vi "CalculateIrradiance.vi"(0 "Base Irradiance µW/cm²":dbl, 1 "Array":dbl[](array[numeric]), 4 "index":i32) -> (5 "Irradiance":dbl, 6 "Base Irradiance Out":dbl, 7 "Array Out":dbl[](array[numeric]))   [LabVIEW 2013]
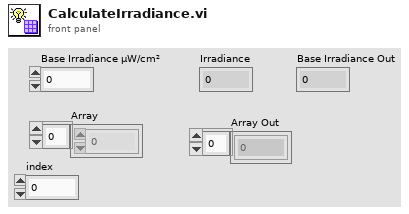
[diagram p1: front panel]
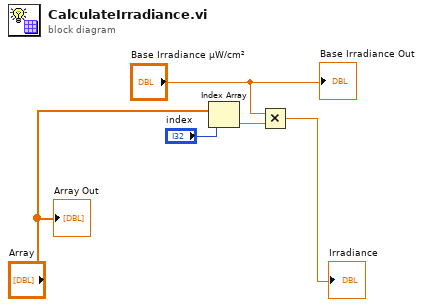
[diagram p0: block diagram]
diagram:
  n1 = Index Array(array="Array", index="index") -> (element=w4:dbl)
  n2 = Multiply(x="Base Irradiance µW/cm²", y=w4) -> (x*y=→"Irradiance":dbl)
  "Array Out" <- "Array"
  "Base Irradiance Out" <- "Base Irradiance µW/cm²"
